vi "Thermal Chamber Controller with Multiple DUT.vi"() -> ()   [LabVIEW 2020]
uses:
  Thermal Chamber Controller/Thermal Chamber Controller.lvclass
  C:/Program Files (x86)/National Instruments/LabVIEW 2020/vi.lib/Asteme/Triarc Framework/Process/Process.lvclass
  C:/Program Files (x86)/National Instruments/LabVIEW 2020/vi.lib/Asteme/Triarc Framework/View/View.lvclass
  Thermal Chamber Controller/Private/Heater State.ctl
  <vilib>/Asteme/Triarc Framework/Process/Process.lvclass/Process.ctl
  <vilib>/Asteme/Triarc Framework/View/View.lvclass/View.ctl
  Device Under Test/Device Under Test.lvclass
  <vilib>/Asteme/Triarc Framework/Process/Protected/Messaging/Enqueue Message.vi
  <vilib>/Asteme/Triarc Framework/View/Public/Get View VI Reference.vi
  <vilib>/Asteme/Triarc Framework/Process/Public/Lifecycle/Get Lifecycle State.vi
  <vilib>/Asteme/Triarc Framework/Process/Private/SubVIs/Wait for finish.vi
  <vilib>/Asteme/Triarc Framework/Process/Private/SubVIs/Set Lifecycle State.vi
  <vilib>/Asteme/Triarc Framework/Process/Protected/Messaging/Request Message.vi
  <vilib>/Utility/error.llb/Clear Errors.vi
  <vilib>/Asteme/Triarc Framework/Process/Private/SubVIs/Enqueue Request Message.vi
  <vilib>/Asteme/Triarc Framework/View/View.lvclass
  <vilib>/Utility/error.llb/Error Cluster From Error Code.vi
  <vilib>/Asteme/Triarc Framework/Process/Private/SubVIs/Wait for Response Message.vi
  <vilib>/Asteme/Triarc Framework/Process/Process.lvclass
  C:/Program Files (x86)/National Instruments/LabVIEW 2020/vi.lib/Asteme/Triarc Framework/Base/Base.lvclass
  C:/Program Files (x86)/National Instruments/LabVIEW 2020/vi.lib/Asteme/Triarc Framework/Error Handler Interface/Error Handler Interface.lvclass
  C:/Program Files (x86)/National Instruments/LabVIEW 2020/vi.lib/Asteme/Triarc Framework/Logging/Logging.lvclass
  C:/Users/anton/Documents/GitHub/Triarc-Examples/Thermal Chamber/Thermal Chamber Controller/Thermal Chamber Controller.lvclass
  C:/Program Files (x86)/National Instruments/LabVIEW 2020/vi.lib/Asteme/Triarc Framework/Helper Loop/Helper Loop.lvclass
  C:/Users/anton/Documents/GitHub/Triarc-Examples/Thermal Chamber/Device Under Test/Device Under Test.lvclass
panel:
  in  "Number of DUTs":i32=5
  out "Self Test Results":bool[](array[boolean])
  # "(The DUT simulator has a self test pass rate of 80%)."
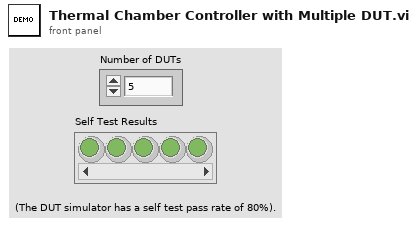
[diagram p1: front panel]
types:
  T1 = typedef "Thermal Chamber Controller.lvclass/Heater State.ctl" = enum16{"Heater Disabled", "Heater Enabled"}
  T2 = typedef "Thermal Chamber Controller.lvclass/Chamber State.ctl" = cluster{"Actual Temperature":dbl, "Temperature Set Point":dbl, "Temperature Ramp Rate":dbl, "Heater State":T1}
  T3 = typedef "Device Under Test.lvclass/Self Test Reply Payload.ctl" = cluster{"Result":bool, "Self Test Error":errorcluster}
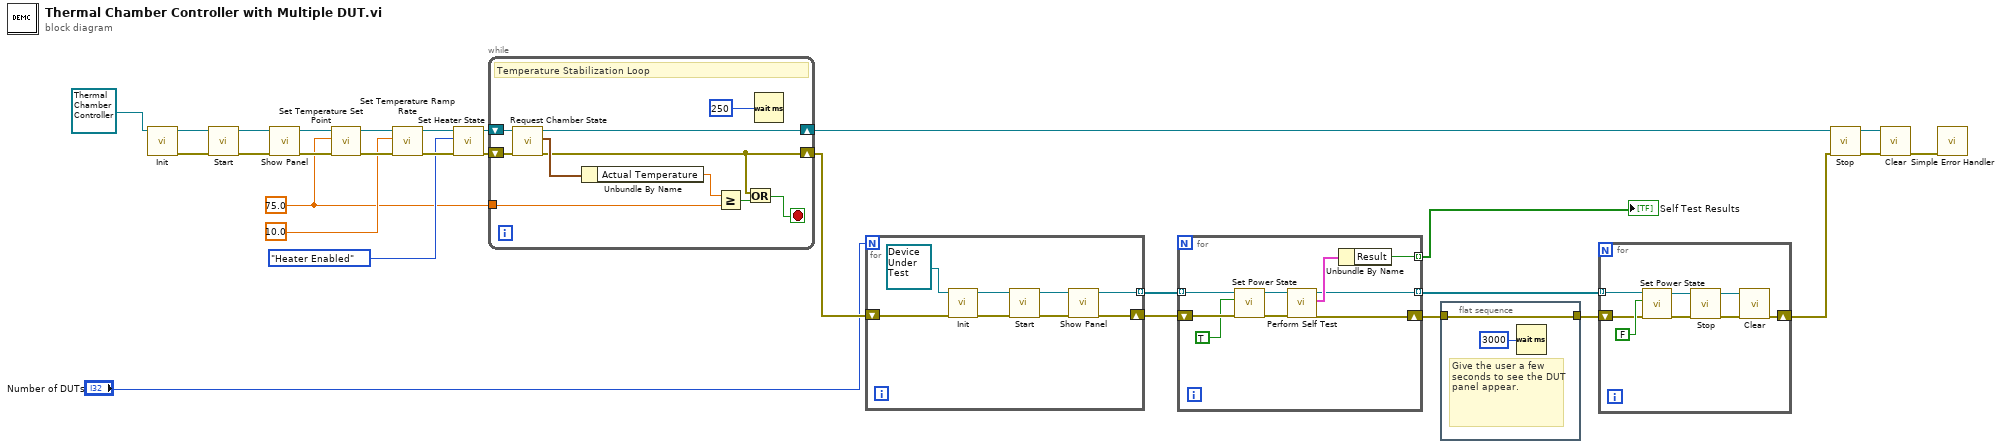
[diagram p0: block diagram]
diagram:
  w11 = 75.0 ("Temperature Set Point")
  n1 = call-dynamic "Init.vi"("View In"=refnum<class "Thermal Chamber Controller.lvclass"> refnum ("Thermal Chamber Controller.lvclass")) -> ("error out"=w28:errorcluster, "View Out"=w29:refnum<class "Thermal Chamber Controller.lvclass">)  [unwired: 9 in]
  n2 = call <vilib>:"Start.vi"("error in (no error)"=w28, "Process In"=w29) -> ("error out"=w27:errorcluster, "Process Out"=w22:refnum<class "Thermal Chamber Controller.lvclass">)  [unwired: 8 in]
  n3 = call <vilib>:"Show Panel.vi"("error in (no error)"=w27, "View In"=w22) -> ("error out"=w23:errorcluster, "View Out"=w20:refnum<class "Thermal Chamber Controller.lvclass">)  [unwired: 8 in]
  n4 = call "Set Temperature Set Point.vi"("error in (no error)"=w23, "Temperature Set Point"=w11, "Thermal Chamber Controller In"=w20) -> ("error out"=w21:errorcluster, "Thermal Chamber Controller Out"=w18:refnum<class "Thermal Chamber Controller.lvclass">)  [unwired: 7 in]
  n5 = call "Set Temperature Ramp Rate.vi"("error in (no error)"=w21, "Temperature Ramp Rate [degC/s]"=10.0, "Thermal Chamber Controller In"=w18) -> ("error out"=w19:errorcluster, "Thermal Chamber Controller Out"=w15:refnum<class "Thermal Chamber Controller.lvclass">)  [unwired: 7 in]
  n6 = call "Set Heater State.vi"("error in (no error)"=w19, "Heater State"=Heater_State."Heater Enabled", "Thermal Chamber Controller In"=w15) -> ("error out"=w16:errorcluster, "Thermal Chamber Controller Out"=w13:refnum<class "Thermal Chamber Controller.lvclass">)  [unwired: 7 in]
  n7 = while {
    shift-right: [w34] -> w8
    shift-left: w16 -> [w39]
    shift-right: [w37] -> w12
    shift-left: w13 -> [w38]
    tunnel: w11 -> [w31]
    stop <- w35 stop-if-true
    # "Temperature Stabilization Loop"
    n8 = call "Request Chamber State.vi"("error in (no error)"=w39, "Thermal Chamber Controller In"=w38) -> ("error out"=w34:errorcluster, "Chamber Status Reply Payload"=w36:T2, "Thermal Chamber Controller Out"=w37:refnum<class "Thermal Chamber Controller.lvclass">)  [unwired: 6 in, 1 out]
    n9 = Unbundle By Name(w36) -> ("Actual Temperature"=w32:dbl)
    n10 = Greater Or Equal?(x=w32, y=w31) -> (x >= y?=w30:bool)
    n11 = Or(x=w34, y=w30) -> (x .or. y?=w35:bool)
    n12 = Wait (ms)(milliseconds to wait=u32 250) -> ()  [unwired: 1 out]
  }
  n13 = for {
    N: "Number of DUTs" -> [_]
    shift-right: [w44] -> w9
    shift-left: w8 -> [w43]
    tunnel: [w45] -> w10 mode=indexing
    n14 = call-dynamic "Init.vi"("error in (no error)"=w43, "View In"=refnum<class "Device Under Test.lvclass"> refnum ("Device Under Test.lvclass")) -> ("error out"=w42:errorcluster, "View Out"=w41:refnum<class "Device Under Test.lvclass">)  [unwired: 8 in]
    n15 = call <vilib>:"Start.vi"("error in (no error)"=w42, "Process In"=w41) -> ("error out"=w46:errorcluster, "Process Out"=w47:refnum<class "Device Under Test.lvclass">)  [unwired: 8 in]
    n16 = call <vilib>:"Show Panel.vi"("error in (no error)"=w46, "View In"=w47) -> ("error out"=w44:errorcluster, "View Out"=w45:refnum<class "Device Under Test.lvclass">)  [unwired: 8 in]
  }
  n17 = for {
    tunnel: w10 -> [w51] mode=indexing
    tunnel: [w55] -> w7 mode=indexing
    tunnel: [w54] -> w4 mode=indexing
    shift-right: [w53] -> w3
    shift-left: w9 -> [w50]
    n18 = call "Set Power State.vi"("error in (no error)"=w50, "Power State"=TRUE, "Device Under Test In"=w51) -> ("error out"=w49:errorcluster, "Device Under Test Out"=w52:refnum<class "Device Under Test.lvclass">)  [unwired: 7 in]
    n19 = call "Perform Self Test.vi"("error in (no error)"=w49, "Device Under Test In"=w52) -> ("error out"=w53:errorcluster, "data"=w56:T3, "Device Under Test Out"=w55:refnum<class "Device Under Test.lvclass">)  [unwired: 6 in, 1 out]
    n20 = Unbundle By Name(w56) -> ("Result"=w54:bool)
  }
  "Self Test Results" <- w4
  n21 = flat-sequence {
    tunnel: w3 -> [w58]
    tunnel: [w58] -> w2
    frame #0 {
      # "Give the user a few seconds to see the DUT panel appear."
      n22 = Wait (ms)(milliseconds to wait=u32 3000) -> ()  [unwired: 1 out]
    }
  }
  n23 = for {
    tunnel: w7 -> [w62] mode=indexing
    shift-right: [w60] -> w6
    shift-left: w2 -> [w59]
    n24 = call "Set Power State.vi"("error in (no error)"=w59, "Power State"=FALSE, "Device Under Test In"=w62) -> ("error out"=w61:errorcluster, "Device Under Test Out"=w63:refnum<class "Device Under Test.lvclass">)  [unwired: 7 in]
    n25 = call <vilib>:"Stop.vi"("error in (no error)"=w61, "Process In"=w63) -> ("error out"=w65:errorcluster, "Process Out"=w64:refnum<class "Device Under Test.lvclass">)  [unwired: 7 in, 1 out]
    n26 = call-dynamic "Clear.vi"("error in (no error)"=w65, "View In"=w64) -> ("error out"=w60:errorcluster)  [unwired: 9 in]
  }
  n27 = call <vilib>:"Stop.vi"("error in (no error)"=w6, "Process In"=w12) -> ("error out"=w25:errorcluster, "Process Out"=w26:refnum<class "Thermal Chamber Controller.lvclass">)  [unwired: 7 in, 1 out]
  n28 = call-dynamic "Clear.vi"("error in (no error)"=w25, "View In"=w26) -> ("error out"=w1:errorcluster)  [unwired: 9 in]
  n29 = call <vilib>:"Simple Error Handler.vi"("error in (no error)"=w1) -> ()  [unwired: 4 in, 5 out]
